vi "Read Acoustic Calibration File.vi"(0 "Cal File Path":path, 11 "error in (no error)":errorcluster) -> (4 "Per Site Acoustic Cal Data":T1[](array[typedef]), 15 "error out":errorcluster)   [LabVIEW 2020]
doc: "Read Acoustic Calibration API reads the calibration data for each site from the input cal file location and returns the data in expected Cal Data format."
uses:
  Acoustic Cal Data Cluster.ctl
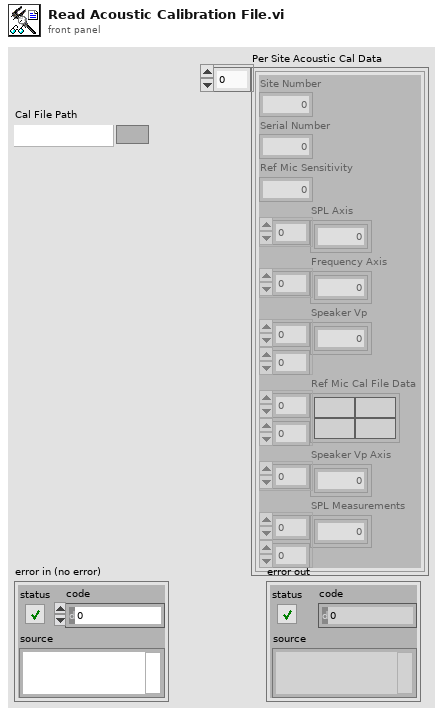
[diagram p1: front panel]
types:
  T1 = typedef "Acoustic Cal Data Cluster.ctl" = cluster{"Site Number":i32, "Serial Number":u32, "Ref Mic Sensitivity":dbl, "SPL Axis":dbl[], "Frequency Axis":dbl[], "Speaker Vp":dbl[][], "Ref Mic Cal File Data":string[][], "Speaker Vp Axis":dbl[], "SPL Measurements":dbl[][]}
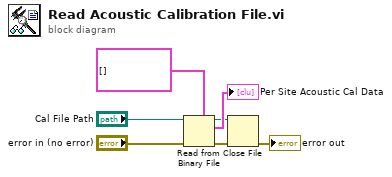
[diagram p0: block diagram]
diagram:
  n1 = Read from Binary File(5:T1[] [] ("Per Site Acoustic Cal Data"), 8:"error in (no error)", 11:"Cal File Path") -> (0:w2:errorcluster, 2:→"Per Site Acoustic Cal Data":T1[], 3:w3:refnum<file>)  [unwired: 3 in, 1 out]
  n2 = Close File(refnum=w3, error in=w2) -> (error out=→"error out":errorcluster)  [unwired: 1 out]
